vi "Update Decay & IRF Parameters Visibility & Caption.vi"(10 "error in (no error)":errorcluster, 11 "Phasor Explorer Decay & IRF Parameters in":refnum<vi>) -> (2 "error out":errorcluster, 3 "Phasor Explorer Decay & IRF Parameters out":refnum<vi>)   [LabVIEW 2019]
uses:
  Phasor Explorer Decay Parameters.ctl
  IRF Model.ctl
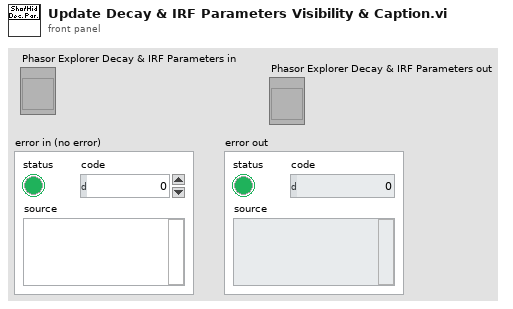
[diagram p1: front panel]
types:
  T1 = typedef "Phasor Explorer Decay Parameters.ctl" = cluster{"Lifetime":dbl[unit], "IRF Offset":dbl[unit], "IRF Period":dbl[unit], "Normalized Decays":bool, "IRF Model":T2, "IRF Parameter 1":dbl[unit]}
  T2 = typedef "IRF Model.ctl" = enum16{"Dirac", "Exponential"}
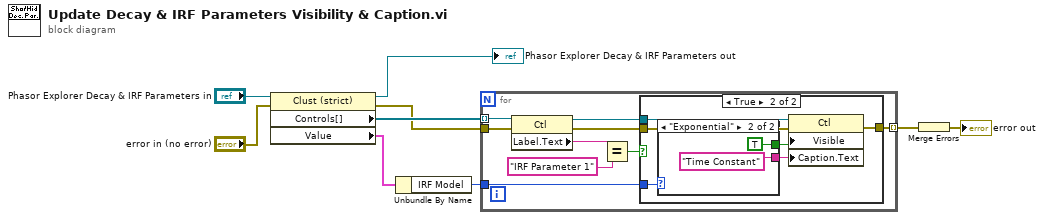
[diagram p0: block diagram]
diagram:
  n1 = property class="Clust (strict)"(reference="Phasor Explorer Decay & IRF Parameters in", error in="error in (no error)") -> (reference out=→"Phasor Explorer Decay & IRF Parameters out":refnum<vi>, error out=w5:errorcluster, "Controls[]"=w6:refnum<vi>[], "Value"=w4:T1)
  n2 = Unbundle By Name(w4) -> ("IRF Model"=w3:T2)
  n3 = for {
    tunnel: w6 -> [w18] mode=indexing
    tunnel: w5 -> [w12]
    tunnel: w3 -> [w11]
    tunnel: [w10] -> w2 mode=indexing
    n4 = property class="Ctl"(reference=w18, error in=w12) -> (reference out=w14:refnum<vi>, error out=w13:errorcluster, "Label.Text"=w17:string)
    n5 = Equal?(x=w17, y="IRF Parameter 1" ("Label.Text")) -> (x = y?=w15:bool)
    n6 = case shown="True" w15 {
      tunnel: w14 -> [_ w25]
      tunnel: w13 -> [w19 w21]
      tunnel: w11 -> [_ w24]
      tunnel: [w19 w20] -> w10
      frame False {
      }
      frame True {
        n7 = case shown="\"Exponential\"" w24 {
          tunnel: [_ TRUE ("Visible")] -> w23
          tunnel: [_ "Time Constant" ("Caption.Text")] -> w22
          frame "Dirac", Default {
          }
          frame "Exponential" {
          }
        }
        n8 = property class="Ctl"(reference=w25, error in=w21, "Visible"=w23, "Caption.Text"=w22) -> (error out=w20:errorcluster)  [unwired: 1 out]
      }
    }
  }
  n9 = Merge Errors(w2) -> (→"error out":errorcluster)
